vi "Histeresis.vi"() -> ()   [LabVIEW 2020]
uses:
  <vilib>/numeric/Random Number (Range) I64.vi
  <vilib>/numeric/sub_Random U32.vi
panel:
  in  "x":dbl
  out "Histeresis":bool
  in  "stop":bool
  out "number":i64
  in  "Min":dbl
  in  "Max":dbl
  out "dentro del rango":bool
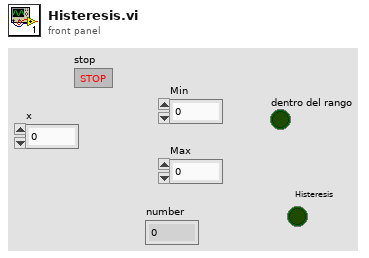
[diagram p1: front panel]
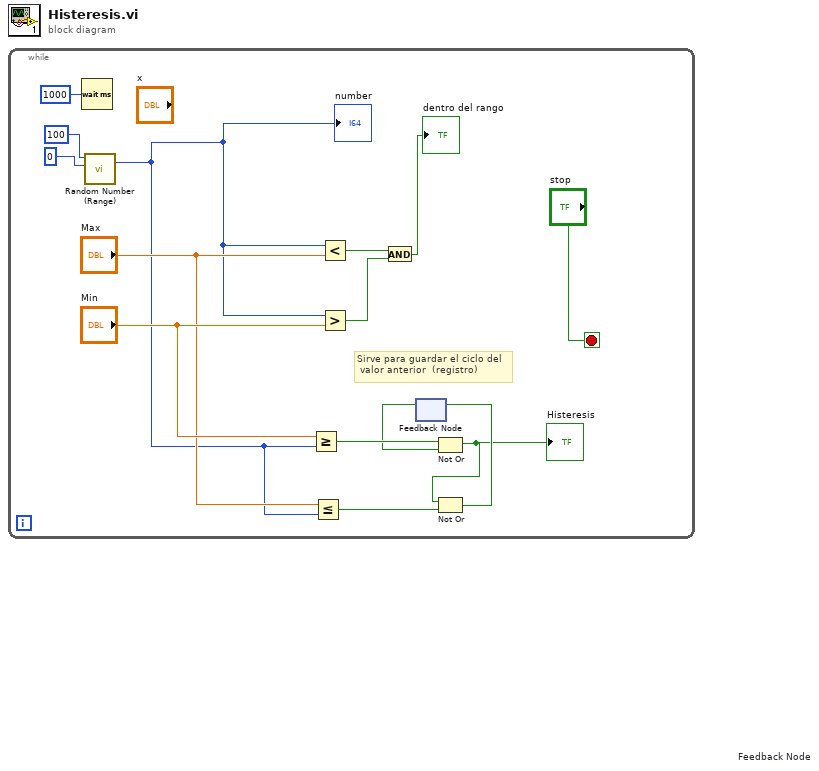
[diagram p0: block diagram]
diagram:
  n1 = while {
    stop <- "stop" stop-if-true
    # "Sirve para guardar el ciclo del\n valor anterior  (registro)"
    n2 = Wait (ms)(milliseconds to wait=u32 1000) -> ()  [unwired: 1 out]
    n3 = call-poly <vilib>:"Random Number (Range).vi"("lower bound (-100)"=u64 0 ("lower bound (0)"), "upper bound (100)"=u64 100) -> ("number"=w1:i64)  [unwired: 9 in]
    "number" <- w1
    n4 = Greater Or Equal?(x="Min", y=w1) -> (x >= y?=w7:bool)
    n5 = Less Or Equal?(x="Max", y=w1) -> (x <= y?=w8:bool)
    n6 = Less?(x=w1, y="Max") -> (x < y?=w10:bool)
    n7 = Greater?(x=w1, y="Min") -> (0:w11:bool)
    n8 = And(x=w10, y=w11) -> (x .and. y?=→"dentro del rango":bool)
    n9 = feedback #1 "Feedback Node"() -> (w6:bool)  [unwired: 1 in]
    n10 = Not Or(1:w6, 2:w7) -> (0:w2:bool)
    "Histeresis" <- w2
    n11 = Not Or(1:w8, 2:w2) -> (0:w5:bool)
    n12 = feedback-in #1(w5) -> ()
  }
